vi "DataSafetyWriteGen.vi"(5 "LastScanPosIn":dbl[](array[numeric]), 7 "XY Graph":T1(array[cluster]), 9 "AllYDataIn":dbl[][](array[numeric]), 11 "error in (no error)":errorcluster) -> (8 "XY Graph Out":T1(array[cluster]), 10 "AllYDataOut":dbl[][](array[numeric]), 15 "error out":errorcluster)   [LabVIEW 2010]
doc: "Ce VI sauvegarde les données d'acquisition pour en garder une copie de sécurité qui peut être rappeller en cas de panne."
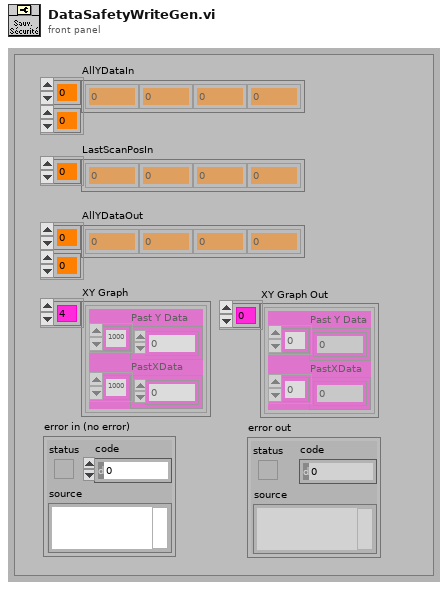
[diagram p1: front panel]
types:
  T1 = cluster{"Past Y Data":dbl[], "PastXData":dbl[]}[]
  T2 = cluster{"AllYDataIn":dbl[][], "XY Graph":cluster{"Past Y Data":dbl[], "PastXData":dbl[]}[], "LastScanPosIn":dbl[]}
  T3 = enum16{"open", "replace", "create", "open or create", "replace or create", "replace or create with confirmation"}
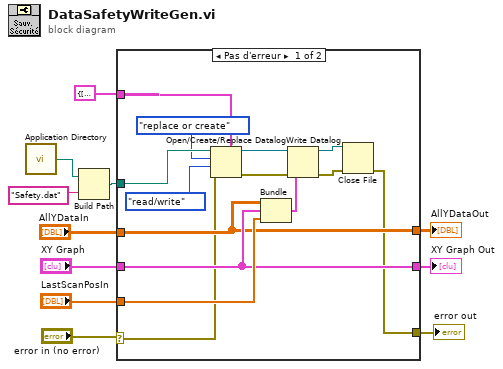
[diagram p0: block diagram]
diagram:
  n1 = call <vilib>:"Application Directory.vi"() -> ("Application Directory"=w1:path)
  n2 = Build Path(base path=w1, name or relative path="Safety.dat") -> (appended path=w2:path)
  n3 = case shown="Pas d'erreur" "error in (no error)" {
    selector: "error in (no error)" -> [w18 w28]
    tunnel: "LastScanPosIn" -> [w25 _]
    tunnel: "AllYDataIn" -> [w23 w27]
    tunnel: "XY Graph" -> [w24 w26]
    tunnel: [w14 w28] -> w7
    tunnel: [w24 w26] -> w6
    tunnel: [w23 w27] -> w5
    tunnel: w2 -> [w22 _]
    tunnel: T2 {"AllYDataIn"=[], "XY Graph"=[], "LastScanPosIn"=[]} -> [w19 _]
    frame No Error {
      n4 = Open/Create/Replace Datalog(5:w19, 8:w18, 9:enum16{"read/write", "read-only", "write-only"}."read/write" ("accès (0 : read/write)"), 10:T3."replace or create" ("opération (0 : open)"), 11:w22) -> (0:w17:errorcluster, 3:w21:refnum<k1>)  [unwired: 1 in, 1 out]
      n5 = Bundle("AllYDataIn"=w23, "XY Graph"=w24, "LastScanPosIn"=w25) -> (w20:T2)  [unwired: 1 in]
      n6 = Write Datalog(4:w17, 6:w20, 7:w21) -> (0:w15:errorcluster, 3:w16:refnum<k1>)
      n7 = Close File(refnum=w16, error in=w15) -> (error out=w14:errorcluster)  [unwired: 1 out]
    }
    frame Error {
    }
  }
  "AllYDataOut" <- w5
  "XY Graph Out" <- w6
  "error out" <- w7
